vi "Main.vi"() -> ()   [LabVIEW 2013]
uses:
  <vilib>/Utility/error.llb/DialogType.ctl
panel:
  in  "выкл.":bool
  in  "IP":string="172.16.21.121"
  in  "SetRemote":bool
  in  "Сброс ERR":bool
  in  "График":bool=TRUE
  in  "Current":u16 caption="мА" max=30 step=1
  in  "SetIB":bool
  in  "Voltage":dbl=0.01 caption="кВ" min=0.01 max=9.9 step=0.1 format="%#.2f"
  in  "SetUB":bool
  out "Режим":bool
  out "Статус":bool
  out "Блокировка":bool
  out "мА":string
  out "Выход":bool
  in  "вкл.":bool
  out "conn src":refnum<k5>
  in  "stop":bool
  out "message":string=" INSTRUCTIONS:\r\rNormal Use:  When using subVIs that incorporate the error in/error out (or error I/O) structure, place this handler where you want to inform the user of an error, typically at the end of the I/O data path, as the last action of the program.  If the error in error? is ERROR, the handler creates a message describing the error and its source.  If the type of dialog = 1 (default), the message is displayed to the user, who can only acknowedge it.  If the type = 2, the user can acknowledge the message or abort execution; aborting a program with active I/O is not recommended.  If the type = 0, no message is displayed; this is used to process the error programmatically, and the error out cluster elements are wired to individual terminals for that reason.  \r\rOther Use:\n\r\nlocal testing.  To test the error code of a subVI or function that does not have the error I/O structure, you can wire its error code and a source string to the local error code and error source inputs.  If error in error? indicates no error and error code is not equal to 0, the local code and source are substituted for the error in values, and error? is set TRUE (ERROR)."
  out "кВ":string
  out "Uвых":dbl(graph)
  # "SPELLMAN 10 кВ 30 мА"
  # "Установки"
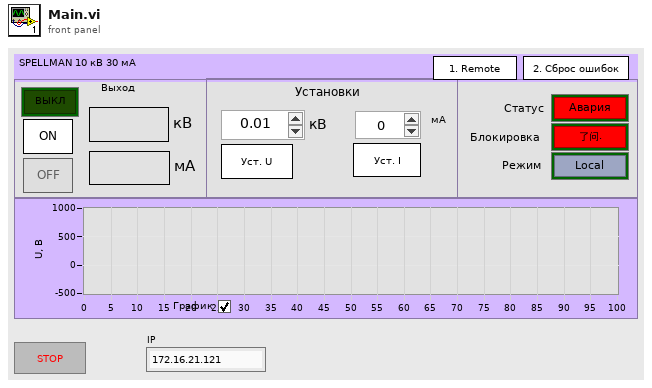
[diagram p1: front panel]
types:
  T1 = typedef "DialogType.ctl" = u16
  T2 = enum8{"Enabled", "Disabled", "Disabled and Grayed Out"}
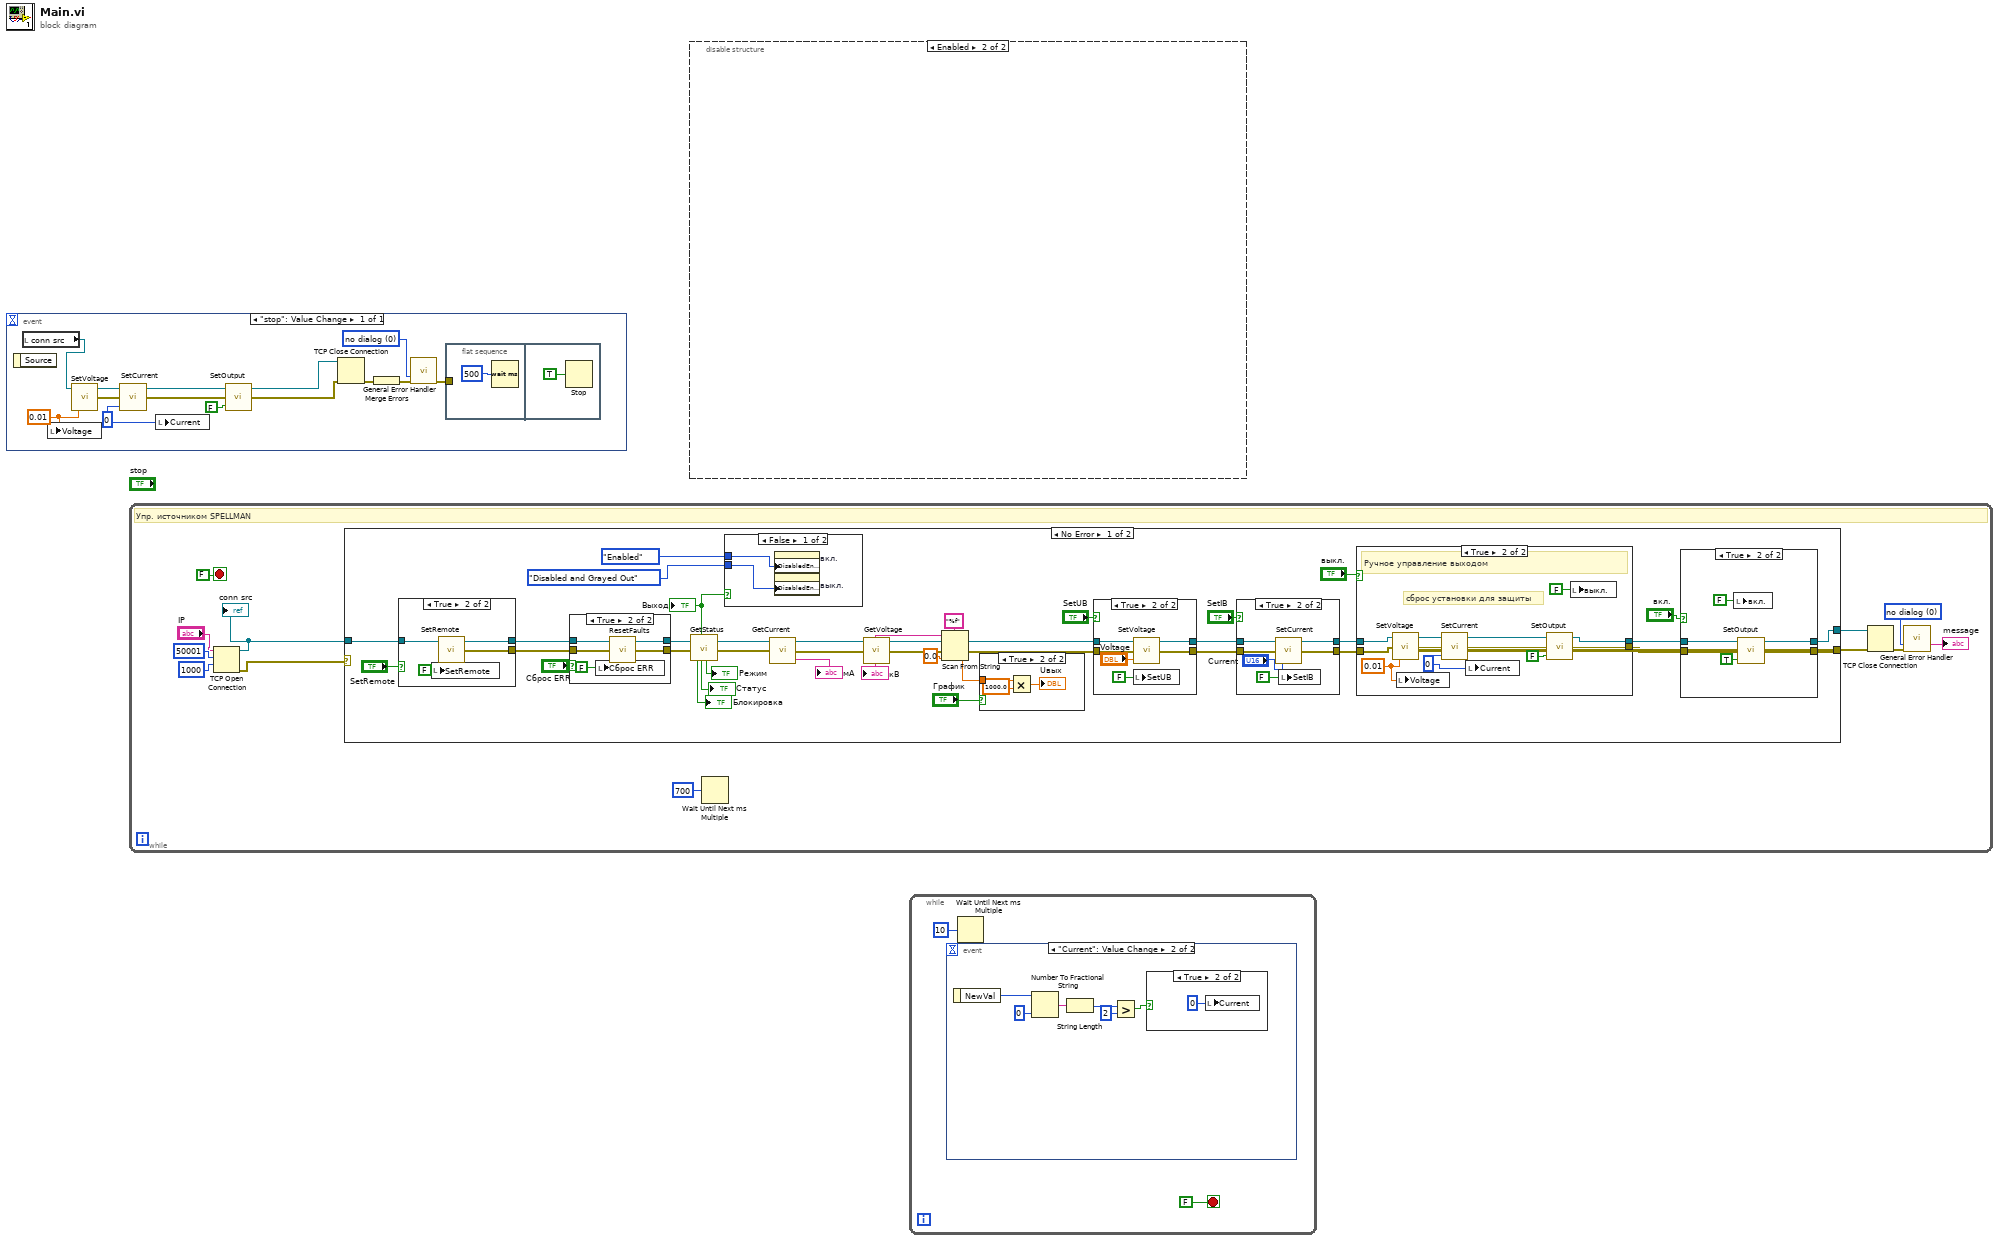
[diagram p0: block diagram]
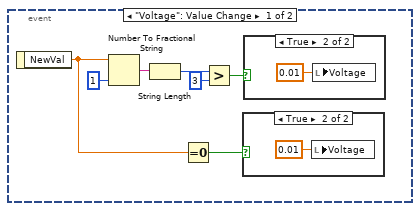
[diagram p2: hidden frame]
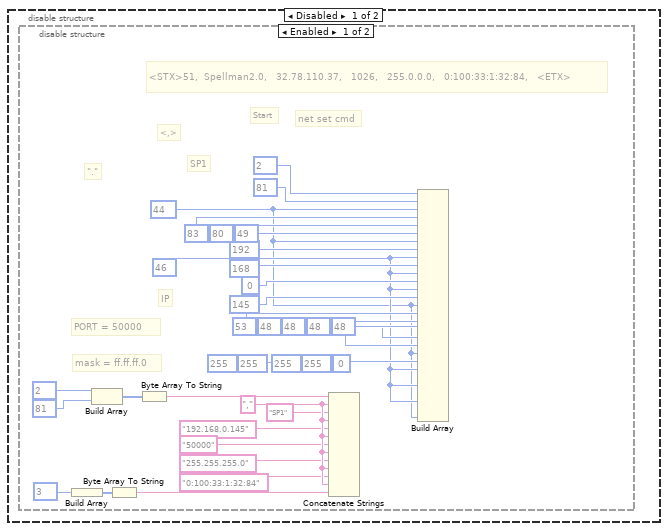
[diagram p6: hidden frame]
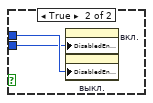
[diagram p8: hidden frame]
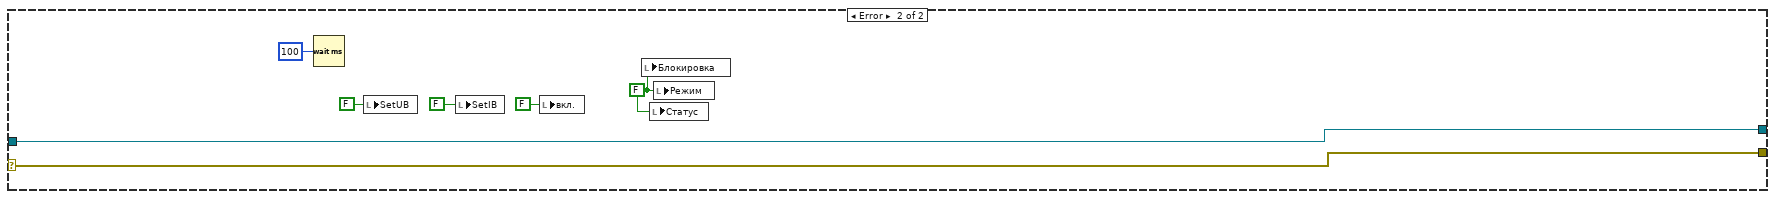
[diagram p16: hidden frame]
diagram:
  n1 = event shown="[0] \"stop\": Value Change" {
    selector: _ -> [_]
    dyn-events: _ -> [_]
    timeout: _ -> [_]
    event "stop": Value Change {
      w1 = u16 0 ("Current")
      w2 = 0.01 ("Voltage")
      w12 = T1 0 items=["no dialog", "OK message", "continue or stop message", "OK message + warnings", "continue/stop + warnings"] ("type of dialog (OK msg:1)")
      n2 = event-data() -> ()  [unwired: 1 in, 1 out]
      n3 = local read "conn src"() -> (w5:refnum<k5>)
      n4 = local write "Voltage"(w2) -> ()
      n5 = call "SetVoltage.vi"("Voltage"=w2, "connection ID"=w5) -> ("error out"=w6:errorcluster, "connection ID out"=w7:refnum<k5>)  [unwired: 1 in, 1 out]
      n6 = call "SetCurrent.vi"("Current"=w1, "error in"=w6, "connection ID in"=w7) -> ("error out"=w8:errorcluster, "connection ID out"=w9:refnum<k5>)  [unwired: 1 out]
      n7 = local write "Current"(w1) -> ()
      n8 = call "SetOutput.vi"("State"=FALSE, "error in"=w8, "connection ID"=w9) -> ("error out"=w3:errorcluster, "connection ID out"=w4:refnum<k5>)  [unwired: 1 in]
      n9 = TCP Close Connection(connection ID=w4, error in (no error)=w3) -> (error out=w14:errorcluster)  [unwired: 1 in, 1 out]
      n10 = Merge Errors(w14) -> (w13:errorcluster)
      n11 = call <vilib>:"General Error Handler.vi"("type of dialog (OK msg:1)"=w12, "error in (no error)"=w13) -> ("error out"=w11:errorcluster)  [unwired: 9 in, 4 out]
      n12 = flat-sequence {
        tunnel: w11 -> [_]
        frame #0 {
          n13 = Wait (ms)(milliseconds to wait=u32 500) -> ()  [unwired: 1 out]
        }
        frame #1 {
          n14 = Stop(stop? (T)=TRUE) -> ()
        }
      }
    }
  }
  n15 = while {
    stop <- FALSE stop-if-true
    w26 = T1 0 items=["no dialog", "OK message", "continue or stop message", "OK message + warnings", "continue/stop + warnings"] ("type of dialog (OK msg:1)")
    # "Упр. источником SPELLMAN"
    n16 = TCP Open Connection(address="IP", remote port or service name=u16 50001 ("Port"), timeout ms (60000)=1000) -> (connection ID=w20:refnum<k5>, error out=w19:errorcluster)  [unwired: 2 in]
    "conn src" <- w20
    n17 = case shown="No Error" w19 {
      selector: w19 -> [_ w128]
      tunnel: w20 -> [w40 w129]
      tunnel: [w34 w129] -> w17
      tunnel: [w33 w128] -> w28
      frame No Error {
        n18 = case shown="True" "SetRemote" {
          tunnel: [w79 w83] -> w41
          tunnel: w40 -> [w79 w82]
          tunnel: [_ w81] -> w39
          frame False {
          }
          frame True {
            n19 = local write "SetRemote"(FALSE ("SetRemote")) -> ()
            n20 = call "SetRemote.vi"("connection ID"=w82) -> ("error out"=w81:errorcluster, "connection ID out"=w83:refnum<k5>)  [unwired: 2 in, 1 out]
          }
        }
        n21 = case shown="True" "Сброс ERR" {
          tunnel: w41 -> [w85 w90]
          tunnel: [w85 w89] -> w42
          tunnel: [w84 w88] -> w43
          tunnel: w39 -> [w84 w86]
          frame False {
          }
          frame True {
            n22 = local write "Сброс ERR"(FALSE ("Сброс ERR")) -> ()
            n23 = call "ResetFaults.vi"("error in"=w86, "connection ID"=w90) -> ("error out"=w88:errorcluster, "connection ID out"=w89:refnum<k5>)  [unwired: 1 in, 1 out]
          }
        }
        n24 = call "GetStatus.vi"("connection ID in"=w42, "error in"=w43) -> ("InterlLoc State"=→"Блокировка":bool, "OutState"=w31:bool, "Fault"=→"Статус":bool, "Rem|Loc"=→"Режим":bool, "connection ID out"=w49:refnum<k5>, "error out"=w48:errorcluster)  [unwired: 12 in]
        "Выход" <- w31
        n25 = case shown="False" w31 {
          tunnel: T2."Enabled" ("Disabled") -> [w68 w70]
          tunnel: T2."Disabled and Grayed Out" ("Disabled") -> [w67 w69]
          frame False {
            n26 = property on="вкл." class="Bool (strict)"("DisabledEnum"=w68) -> ()  [unwired: 2 in, 2 out]
            n27 = property on="выкл." class="Bool (strict)"("DisabledEnum"=w67) -> ()  [unwired: 2 in, 2 out]
          }
          frame True {
            n28 = property on="вкл." class="Bool (strict)"("DisabledEnum"=w69) -> ()  [unwired: 2 in, 2 out]
            n29 = property on="выкл." class="Bool (strict)"("DisabledEnum"=w70) -> ()  [unwired: 2 in, 2 out]
          }
        }
        n30 = call "GetCurrent.vi"("error in"=w48, "connection ID"=w49) -> ("Current"=→"мА":string, "error out"=w66:errorcluster, "connection ID out"=w65:refnum<k5>)  [unwired: 1 out]
        n31 = call "GetVoltage.vi"("error in"=w66, "connection ID"=w65) -> ("Voltage"=w60:string, "error out"=w57:errorcluster, "connection ID out"=w64:refnum<k5>)  [unwired: 1 out]
        "кВ" <- w60
        n32 = Scan From String(format string="%f", input string=w60, error in=w57, default 1=0.0 ("default (0 I32)")) -> (error out=w56:errorcluster, output 1=w58:dbl)  [unwired: 1 in, 2 out]
        n33 = case shown="True" "График" {
          tunnel: w58 -> [_ w91]
          frame False {
          }
          frame True {
            n34 = Multiply(x=w91, y=1000.0) -> (x*y=→"Uвых":dbl)
          }
        }
        n35 = case shown="True" "SetUB" {
          tunnel: w56 -> [w103 w109]
          tunnel: [w103 w108] -> w53
          tunnel: w64 -> [w102 w107]
          tunnel: [w102 w105] -> w54
          frame False {
          }
          frame True {
            n36 = call "SetVoltage.vi"("Voltage"="Voltage", "error in"=w109, "connection ID"=w107) -> ("error out"=w108:errorcluster, "connection ID out"=w105:refnum<k5>)  [unwired: 1 out]
            n37 = local write "SetUB"(FALSE ("SetUB")) -> ()
          }
        }
        n38 = case shown="True" "SetIB" {
          tunnel: w54 -> [w95 w100]
          tunnel: w53 -> [w94 w99]
          tunnel: [w94 w98] -> w52
          tunnel: [w95 w97] -> w51
          frame False {
          }
          frame True {
            n39 = call "SetCurrent.vi"("Current"="Current", "error in"=w99, "connection ID in"=w100) -> ("error out"=w98:errorcluster, "connection ID out"=w97:refnum<k5>)  [unwired: 1 out]
            n40 = local write "SetIB"(FALSE ("SetUB")) -> ()
          }
        }
        n41 = case shown="True" "выкл." {
          tunnel: [w111 w115] -> w37
          tunnel: [w110 w116] -> w32
          tunnel: w52 -> [w110 w118]
          tunnel: w51 -> [w111 w117]
          frame False {
          }
          frame True {
            w113 = u16 0 ("Current")
            w114 = 0.01 ("Voltage")
            # "сброс установки для защиты"
            # "Ручное управление выходом"
            n42 = call "SetVoltage.vi"("Voltage"=w114, "error in"=w118, "connection ID"=w117) -> ("error out"=w119:errorcluster, "connection ID out"=w120:refnum<k5>)  [unwired: 1 out]
            n43 = local write "Voltage"(w114) -> ()
            n44 = call "SetCurrent.vi"("Current"=w113, "error in"=w119, "connection ID in"=w120) -> ("error out"=w121:errorcluster, "connection ID out"=w122:refnum<k5>)  [unwired: 1 out]
            n45 = local write "Current"(w113) -> ()
            n46 = call "SetOutput.vi"("State"=FALSE, "error in"=w121, "connection ID"=w122) -> ("error out"=w116:errorcluster, "connection ID out"=w115:refnum<k5>)  [unwired: 1 in]
            n47 = local write "выкл."(FALSE ("выкл.")) -> ()
          }
        }
        n48 = case shown="True" "вкл." {
          tunnel: w37 -> [w72 w78]
          tunnel: [w72 w77] -> w34
          tunnel: [w71 w76] -> w33
          tunnel: w32 -> [w71 w75]
          frame False {
          }
          frame True {
            n49 = local write "вкл."(FALSE ("вкл.")) -> ()
            n50 = call "SetOutput.vi"("State"=TRUE, "error in"=w75, "connection ID"=w78) -> ("error out"=w76:errorcluster, "connection ID out"=w77:refnum<k5>)  [unwired: 1 in]
          }
        }
      }
      frame Error {
        w124 = FALSE ("Режим")
        n51 = Wait (ms)(milliseconds to wait=u32 100) -> ()  [unwired: 1 out]
        n52 = local write "SetUB"(FALSE ("SetUB")) -> ()
        n53 = local write "SetIB"(FALSE ("SetUB")) -> ()
        n54 = local write "вкл."(FALSE ("вкл.")) -> ()
        n55 = local write "Блокировка"(w124) -> ()
        n56 = local write "Статус"(w124) -> ()
        n57 = local write "Режим"(w124) -> ()
      }
    }
    n58 = Wait Until Next ms Multiple(millisecond multiple=u32 700 ("milliseconds to wait")) -> ()  [unwired: 1 out]
    n59 = TCP Close Connection(connection ID=w17, error in (no error)=w28) -> (error out=w27:errorcluster)  [unwired: 2 out]
    n60 = call <vilib>:"General Error Handler.vi"("type of dialog (OK msg:1)"=w26, "error in (no error)"=w27) -> ("message"=→"message":string)  [unwired: 9 in, 4 out]
  }
  n61 = disable-structure shown="Enabled" {
    frame Disabled {
      n62 = disable-structure shown="Enabled" {
        frame Enabled {
          w140 = "," ("string")
          (unwired) u8 0 ("y")
          (unwired) u8 255 ("y")
          (unwired) u8 255 ("y")
          (unwired) u8 255 ("y")
          w145 = u8 46 ("y")
          w144 = u8 44 ("y")
          # "mask = ff.ff.ff.0"
          # "PORT = 50000"
          # "IP"
          # "\".\""
          # "net set cmd"
          # "Start"
          # "<,>"
          # "SP1"
          # "<STX>51,  Spellman2.0,   32.78.110.37,   1026,   255.0.0.0,   0:100:33:1:32:84,   <ETX>"
          n63 = Build Array(u8 3 ("y")) -> (w142:u8[])
          n64 = Build Array(u8 2 ("y"), u8 81 ("y")) -> (w131:u8[])
          n65 = Byte Array To String(unsigned byte array=w142) -> (string=w143:string)
          n66 = Byte Array To String(unsigned byte array=w131) -> (string=w134:string)
          n67 = Concatenate Strings(w134, w140, "SP1" ("string"), w140, "192.168.0.145", w140, "50000", w140, "255.255.255.0", w140, "0:100:33:1:32:84", w140, w143) -> ()  [unwired: 1 out]
          n68 = Build Array(u8 2 ("y"), u8 81 ("y"), w144, u8 83 ("y"), u8 80 ("y"), u8 49 ("y"), w144, u8 192 ("y"), w145, u8 168 ("y"), w145, u8 0 ("y"), w145, u8 145 ("y"), w144, u8 53 ("y"), u8 48 ("y"), u8 48 ("y"), u8 48 ("y"), u8 48 ("y"), w144, u8 255 ("y"), w145, w145, w145, w144) -> ()  [unwired: 3 in, 1 out]
        }
        frame Disabled {
        }
      }
    }
    frame Enabled {
    }
  }
  n69 = while {
    stop <- FALSE stop-if-true
    n70 = event shown="[1] \"Current\": Value Change" {
      selector: _ -> [_ _]
      dyn-events: _ -> [_ _]
      timeout: _ -> [_ _]
      event "Voltage": Value Change {
        n71 = event-data() -> ("NewVal"=w164:dbl)  [unwired: 1 in]
        n72 = Number To Fractional String(number=w164, precision (6)=i16 1) -> (F-format string=w168:string)  [unwired: 2 in]
        n73 = String Length(string=w168) -> (length=w167:i32)
        n74 = Equal To 0?(x=w164) -> (x = 0?=w163:bool)
        n75 = Greater?(x=w167, y=3) -> (0:w165:bool)
        n76 = case shown="True" w163 {
          frame False {
          }
          frame True {
            n77 = local write "Voltage"(0.01 ("Voltage")) -> ()
          }
        }
        n78 = case shown="True" w165 {
          frame False {
          }
          frame True {
            n79 = local write "Voltage"(0.01 ("Voltage")) -> ()
          }
        }
      }
      event "Current": Value Change {
        n80 = event-data() -> ("NewVal"=w177:u16)  [unwired: 1 in]
        n81 = Number To Fractional String(number=w177, precision (6)=i16 0) -> (F-format string=w175:string)  [unwired: 2 in]
        n82 = String Length(string=w175) -> (length=w174:i32)
        n83 = Greater?(x=w174, y=2) -> (0:w172:bool)
        n84 = case shown="True" w172 {
          frame False {
          }
          frame True {
            n85 = local write "Current"(u16 0 ("Voltage")) -> ()
          }
        }
      }
    }
    n86 = Wait Until Next ms Multiple(millisecond multiple=u32 10 ("milliseconds to wait")) -> ()  [unwired: 1 out]
  }
